vi "Adjust LoadSensor Cal.vi"(10 "0_Load":dbl, 11 "LS CalData In":dbl[](array[numeric])) -> (3 "LS CalData Out":dbl[](array[numeric]))   [LabVIEW 2015]
uses:
  Controls/Gen2 FT Globals.vi
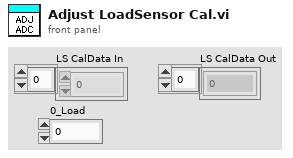
[diagram p1: front panel]
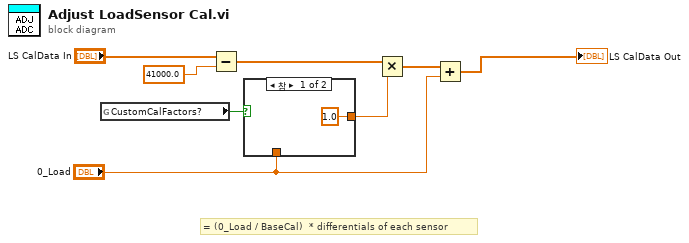
[diagram p0: block diagram]
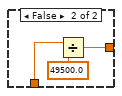
[diagram p2: hidden frame]
diagram:
  # "= (0_Load / BaseCal)  * differentials of each sensor"
  n1 = global read "Gen2 FT Globals.vi" "CustomCalFactors?"() -> (w1:bool)
  n2 = Subtract(x="LS CalData In", y=41000.0) -> (x-y=w4:dbl[])
  n3 = case shown="참" w1 {
    tunnel: "0_Load" -> [_ w12]
    tunnel: [1.0 w10] -> w3
    frame True {
    }
    frame False {
      n4 = Divide(x=w12, y=49500.0) -> (x/y=w10:dbl)
    }
  }
  n5 = Multiply(x=w4, y=w3) -> (x*y=w5:dbl[])
  n6 = Add(x=w5, y="0_Load") -> (x+y=→"LS CalData Out":dbl[])
